vi "Unflatten.vi"(8 "error in (no error)":errorcluster, 11 "Wavelength iHR320 in":refnum<class "Wavelength iHR320.lvclass">) -> (0 "error out":errorcluster, 3 "Wavelength iHR320 out":refnum<class "Wavelength iHR320.lvclass">)   [LabVIEW 2009, in "Wavelength iHR320.lvclass"]
uses:
  Wavelength iHR320.lvclass
  Scanner/Scanner.lvclass
  Global/File Locations.vi
  Wavelength iHR320.lvclass/Wavelength iHR320.ctl
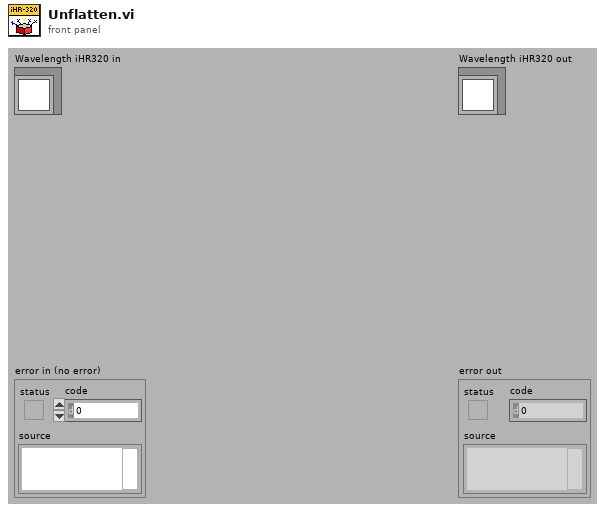
[diagram p1: front panel]
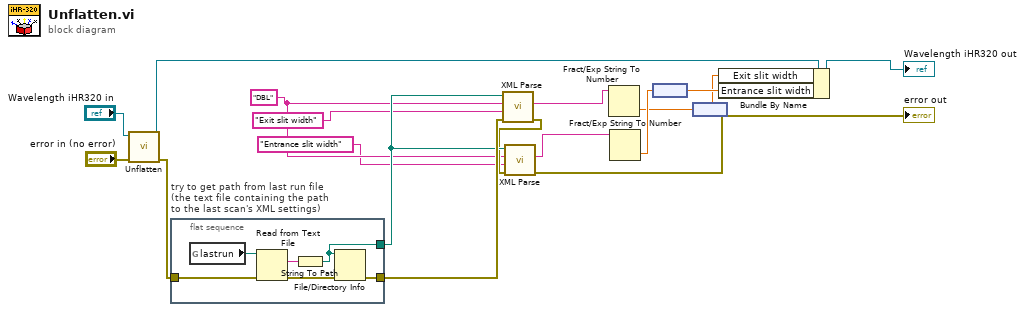
[diagram p0: block diagram]
diagram:
  w9 = "DBL"
  n1 = call-parent "Unflatten.vi"("error in (no error)"="error in (no error)", "Scanner in"="Wavelength iHR320 in") -> ("error out"=w14:errorcluster, "Scanner out"=w18:refnum<class "Wavelength iHR320.lvclass">)  [unwired: 8 in]
  n2 = flat-sequence "try to get path from last run file\n(the text file containing the path\nto the last scan's XML settings)" {
    tunnel: [w24] -> w12
    tunnel: [w20] -> w13
    tunnel: w14 -> [w19]
    frame #0 {
      n3 = global read "File Locations.vi" "lastrun"() -> (w22:path)
      n4 = Read from Text File(file (use dialog)=w22, error in=w19) -> (text=w23:string, error out=w21:errorcluster)  [unwired: 4 out]
      n5 = String To Path(string=w23) -> (path=w24:path)
      n6 = File/Directory Info(path=w24, error in=w21) -> (error out=w20:errorcluster)  [unwired: 6 out]
    }
  }
  n7 = call "XML Parse.vi"("error in (no error)"=w13, "Name String"="Exit slit width", "Type String"=w9, "Path"=w12) -> ("error out"=w11:errorcluster, "String Out"=w3:string)  [unwired: 6 in]
  n8 = call "XML Parse.vi"("error in (no error)"=w11, "Name String"="Entrance slit width", "Type String"=w9, "Path"=w12) -> ("error out"=→"error out":errorcluster, "String Out"=w6:string)  [unwired: 6 in]
  n9 = Fract/Exp String To Number(string=w3) -> (number=w2:dbl)  [unwired: 3 in, 1 out]
  n10 = Fract/Exp String To Number(string=w6) -> (number=w5:dbl)  [unwired: 3 in, 1 out]
  n11 = node(w5) -> (w4:dbl[unit])
  n12 = node(w2) -> (w1:dbl[unit])
  n13 = Bundle By Name(cluster=w18, "Exit slit width"=w1, "Entrance slit width"=w4) -> (→"Wavelength iHR320 out":refnum<class "Wavelength iHR320.lvclass">)
